vi "Continuity.vi"(0 "TSM context":T4, 5 "Supply Pins and Current Limits (set to 0V)":T1[](array[typedef]) {"Current Limit (A)" format="%#_13p"}, 7 "Continuity Test Pins and Current Levels":T3[](array[typedef]) {"Current Level (A)" format="%#_13p"}, 9 "Continuity Test Pins Configuration":T2={"DCPower Pins Voltage Limit (V)"=1.0, "Digital Pins Voltage Limit High (V)"=2.5, "Digital Pins Voltage Limit Low (V)"=-1.5, "Aperture Time (s)"=4e-06, "Settling Time (s)"=0.0005} {"Settling Time (s)" format="%#_13p"; "Aperture Time (s)" format="%#_13p"; "Digital Pins Voltage Limit Low (V)" format="%#_13p"; "Digital Pins Voltage Limit High (V)" format="%#_13p"; "DCPower Pins Voltage Limit (V)" format="%#_13p"}) -> (15 "error out":errorcluster)   [LabVIEW 2020]
doc: "This VI tests continuity on all DCPower or Digital pins specified in the input array. Continuity is tested serially for each pin by forcing the requested Test Level current, measuring and publishing the resulting voltage, and then forcing 0V on that line."
uses:
  <vilib>/NI_TestStand_SemiconductorModule/NI_TestStand_Semiconductor_Module.lvlibp/PinMap/General/SemiconductorModuleContext.ctl
  Typedefs/Continuity Test Pins.ctl
  Typedefs/Continuity Test Pins Configuration.ctl
  Typedefs/Continuity Test Supply Pins.ctl
  <vilib>/NI_TestStand_SemiconductorModule/NI_TestStand_Semiconductor_Module.lvlibp/PinMap/General/NIInstrumentTypeIDs.ctl
  <instrlib>/niDCPower/nidcpower.llb/niDCPower Sense.ctl
  <instrlib>/niDCPower/nidcpower.llb/niDCPower Wait For Event - Event.ctl
  69e15daa-21bc-4a86-876e-45ae4f872e77.vi
  7341af22-bb1b-4db6-ae5f-e70a74fc99ec.vi
  3f155922-c876-4283-947d-51e7db997094.vi
  cab31188-4031-40a5-8ba5-f7a05916ad31.vi
  4e72e363-04f0-4c76-a5e4-36f1355fad37.vi
  4a7f1c6e-2141-4ac2-bcbe-4ddac98e05b0.vi
  69e15daa-21bc-4a86-876e-45ae4f872e77.vi/37e36e8e-52ea-454a-87f9-b48a49eb94f9.vi
  69e15daa-21bc-4a86-876e-45ae4f872e77.vi/7a476e54-2186-4dad-b590-ad3942d096a6.vi
  69e15daa-21bc-4a86-876e-45ae4f872e77.vi/0fe00e69-3e59-4a7f-af61-7afbdd073a88.vi
  69e15daa-21bc-4a86-876e-45ae4f872e77.vi/e6b7bfbe-abe8-4733-8e43-b833ff7e14d5.vi
  7341af22-bb1b-4db6-ae5f-e70a74fc99ec.vi/e13535e0-0cde-4935-b31f-df609d882bf7.vi
  7341af22-bb1b-4db6-ae5f-e70a74fc99ec.vi/3a3479db-a9d1-451a-bc22-44f502cf356f.vi
  7341af22-bb1b-4db6-ae5f-e70a74fc99ec.vi/989d4714-5b7c-4079-81e3-211be10dc077.vi
  7341af22-bb1b-4db6-ae5f-e70a74fc99ec.vi/1a487ccc-7edf-462f-8e0a-db08c9486ef7.vi
  7341af22-bb1b-4db6-ae5f-e70a74fc99ec.vi/c9d031c9-6d94-47b7-9259-545c97247752.vi
  3f155922-c876-4283-947d-51e7db997094.vi/b53c6634-6278-4ab4-ad22-deef7c3257c8.vi
  3f155922-c876-4283-947d-51e7db997094.vi/c97d13a2-db54-44f2-8789-f416a58a5b16.vi
  3f155922-c876-4283-947d-51e7db997094.vi/975b8a18-37a4-405e-b68c-dfb8626d50ee.vi
  3f155922-c876-4283-947d-51e7db997094.vi/86300431-e79c-44d5-990a-071b252c0ae5.vi
  cab31188-4031-40a5-8ba5-f7a05916ad31.vi/9ed1208e-9e24-434b-9077-fc28cb587a19.vi
  cab31188-4031-40a5-8ba5-f7a05916ad31.vi/8ec5e351-fcbd-491e-9dc1-09518d2cf07d.vi
  cab31188-4031-40a5-8ba5-f7a05916ad31.vi/9a5011c0-d40c-4ff4-90a3-5e05d61ad4c8.vi
  cab31188-4031-40a5-8ba5-f7a05916ad31.vi/d089af44-28b1-43b8-9543-ae158de0acbd.vi
  4e72e363-04f0-4c76-a5e4-36f1355fad37.vi/ca0fc33b-5c63-48b0-b4a8-701cf7564698.vi
  4e72e363-04f0-4c76-a5e4-36f1355fad37.vi/d07ff0df-60b4-435a-afe9-5c803e6a7680.vi
  4e72e363-04f0-4c76-a5e4-36f1355fad37.vi/0037e193-eb15-4f67-9373-277439ca96e3.vi
  4e72e363-04f0-4c76-a5e4-36f1355fad37.vi/04a00edb-35d4-47ed-b21f-d8dfa56efb37.vi
  Common/Instrument Control/Digital/SubVIs/SSC Digital Calculate Per-Site Per-Pin to Per-Instrument LUT.vi
  4a7f1c6e-2141-4ac2-bcbe-4ddac98e05b0.vi/7ab91422-1a66-4814-9877-4eb2634f872c.vi
  4a7f1c6e-2141-4ac2-bcbe-4ddac98e05b0.vi/78867d26-a5ff-4ac0-84e1-08aa210c9386.vi
  3f155922-c876-4283-947d-51e7db997094.vi/86300431-e79c-44d5-990a-071b252c0ae5.vi/8c0f5037-9bd0-4b91-af38-cdea4b9b3604.vi
  Common/Instrument Control/Shared SubVIs/Trim Whitespace [Inlined].vi
  Common/Instrument Control/DCPower/SubVIs/SSC DCPower Expanded Pin List to SSC Index.vi
  Common/Instrument Control/Shared SubVIs/Channel List to Pins.vi
  <vilib>/NI_TestStand_SemiconductorModule/NI_TestStand_Semiconductor_Module.lvlibp/PinMap/PinQueryContext/MultiplePinMultipleSessionQueryContext/MultiplePinMultipleSessionQueryContext.lvclass
  C:/Program Files/National Instruments/LabVIEW 2020/vi.lib/NI_TestStand_SemiconductorModule/NI_TestStand_Semiconductor_Module.lvlibp/PinMap/PinQueryContext/PinQueryContext.lvclass
  <vilib>/NI_TestStand_SemiconductorModule/NI_TestStand_Semiconductor_Module.lvlibp/PinMap/Digital Pattern/PinQueryContext/DigitalPatternPinQueryContext.lvclass
  C:/Program Files/National Instruments/LabVIEW 2020/vi.lib/NI_TestStand_SemiconductorModule/NI_TestStand_Semiconductor_Module.lvlibp/PinMap/PinQueryContext/MultipleSessionPinQueryContext.lvclass
  Common/Instrument Control/Digital/SSC Digital/PPMU/SSC Digital PPMU Source Voltage.vi
  Common/Instrument Control/DCPower/SSC DCPower/Source/Constant Voltage/SSC DCPower Force Voltage Array Symmetric Limits.vi
  Common/Instrument Control/DCPower/SSC DCPower/SSC DCPower Configure Measurements.vi
  Common/Instrument Control/DCPower/SSC DCPower/Measure/SSC DCPower Configure Settings Array.vi
  <vilib>/Utility/error.llb/Error Cluster From Error Code.vi
  Common/Instrument Control/Digital/SSC Digital/PPMU/SSC Digital PPMU Configure Voltage Limits.vi
  Common/Instrument Control/Digital/SSC Digital/PPMU/SSC Digital PPMU Configure Aperture Time.vi
  Common/Instrument Control/DCPower/SSC DCPower/Source/Constant Current/SSC DCPower Force Current Array Symmetric Limits.vi
  Common/Instrument Control/DCPower/SSC DCPower/Triggers and Events/SSC DCPower Wait for Event.vi
  Common/Instrument Control/DCPower/SSC DCPower/SSC DCPower Measure.vi
  <vilib>/NI_TestStand_SemiconductorModule/NI_TestStand_Semiconductor_Module.lvlibp/PinMap/General/Publish/PublishDataDouble1D.vi
  Common/Instrument Control/Digital/SSC Digital/PPMU/SSC Digital PPMU Source Current.vi
  <vilib>/NI_TestStand_SemiconductorModule/NI_TestStand_Semiconductor_Module.lvlibp/PinMap/General/Publish/PublishDataDouble2D.vi
  <vilib>/NI_TestStand_SemiconductorModule/NI_TestStand_Semiconductor_Module.lvlibp
  C:/Program Files/National Instruments/LabVIEW 2020/vi.lib/NI_TestStand_SemiconductorModule/NI_TestStand_Semiconductor_Module.lvlibp/PinMap/PinQueryContext/MultiplePinMultipleSessionQueryContext/MultiplePinMultipleSessionQueryContext.lvclass
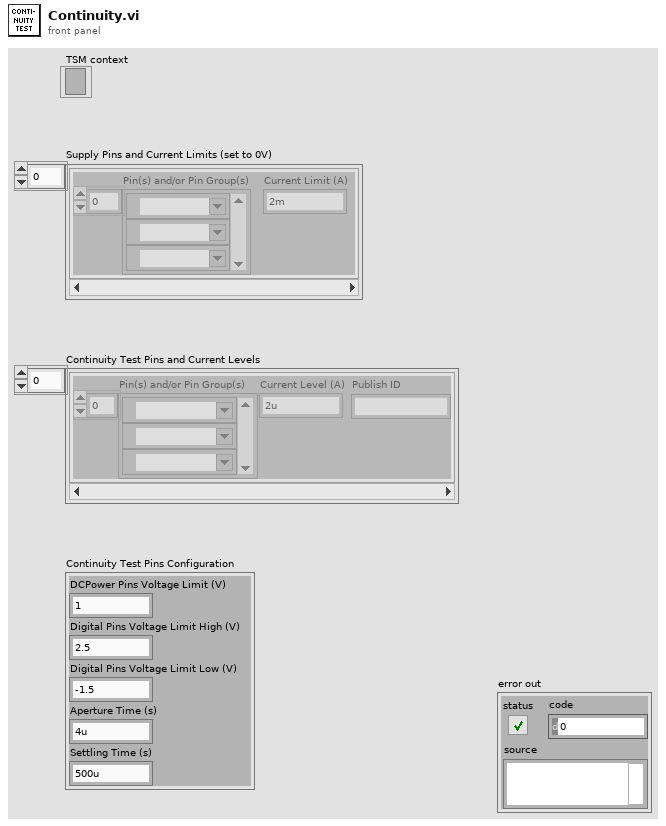
[diagram p1: front panel]
types:
  T1 = typedef "Continuity Test Supply Pins.ctl" = cluster{"Pin(s) and/or Pin Group(s)":tag[], "Current Limit (A)":dbl}
  T2 = typedef "Continuity Test Pins Configuration.ctl" = cluster{"DCPower Pins Voltage Limit (V)":dbl, "Digital Pins Voltage Limit High (V)":dbl, "Digital Pins Voltage Limit Low (V)":dbl, "Aperture Time (s)":dbl, "Settling Time (s)":dbl}
  T3 = typedef "Continuity Test Pins.ctl" = cluster{"Pin(s) and/or Pin Group(s)":tag[], "Current Level (A)":dbl, "Publish ID":string}
  T4 = typedef "NI_TestStand_Semiconductor_Module.lvlibp/SemiconductorModuleContext.ctl" = refnum<k7>
  T5 = cluster{"Site Numbers":i32[], "DCPower Test Levels (A)":dbl[], "DCPower Test Pins":tag[], "DCPower Publish IDs":tag[], "Digital Test Levels (A)":dbl[], "Digital Test Pins":tag[], "Digital Publish IDs":tag[], "Digital Current Range (A)":dbl}
  T6 = typedef "NI_TestStand_Semiconductor_Module.lvlibp/NIInstrumentTypeIDs.ctl" = string
  T7 = typedef "NI_TestStand_Semiconductor_Module.lvlibp/TSM_Pin.ctl" = tag
  T8 = typedef "TSM SSC Digital.ctl" = cluster{"Pin Query Context":refnum<class "DigitalPatternPinQueryContext.lvclass">, "SSC":T9[], "Site Numbers":i32[], "Pins":tag[]}
  T9 = typedef "SSC Digital.ctl" = cluster{"Session":refnum<k15>, "Channel List":string, "Site List":string}
  T10 = typedef "TSM SSC DCPower.ctl" = cluster{"Pin Query Context":refnum<class "MultiplePinMultipleSessionQueryContext.lvclass">, "SSC":T11[], "Site Numbers":i32[], "Pins":T12[], "Pins Expanded":T14[]}
  T11 = typedef "SSC DCPower.ctl" = cluster{"Session":refnum<k15>, "Chan":string, "Channel List":string}
  T12 = typedef "TSM Pin Information.ctl" = cluster{"Pin":tag, "Type":T13, "Count":i32}
  T13 = typedef "TSM Pin Type Identifier.ctl" = enum8{"DUT Pin", "System Pin", "Pin Group", "Not Determined"}
  T14 = typedef "TSM Expanded Pin Information.ctl" = cluster{"Pin":tag, "Type":T13, "Index":i32}
  T15 = typedef "niDCPower Sense.ctl" = i32
  T16 = typedef "niDCPower Wait For Event - Event.ctl" = i32
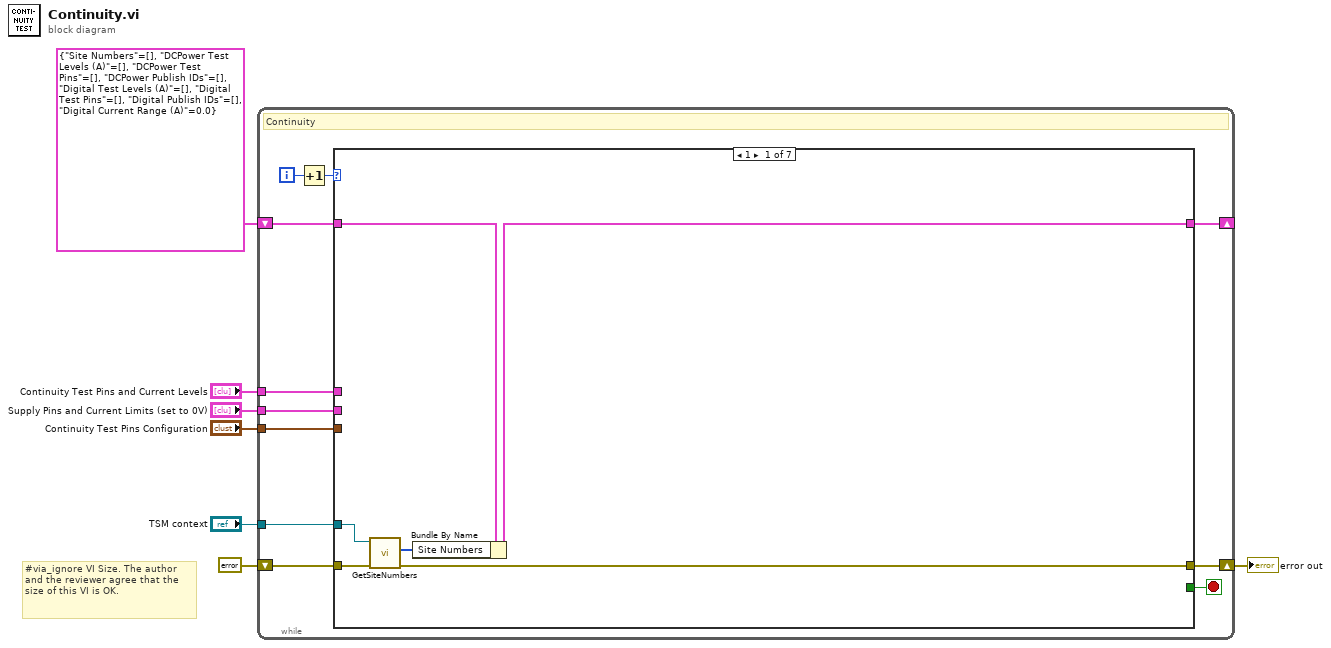
[diagram p0: block diagram]
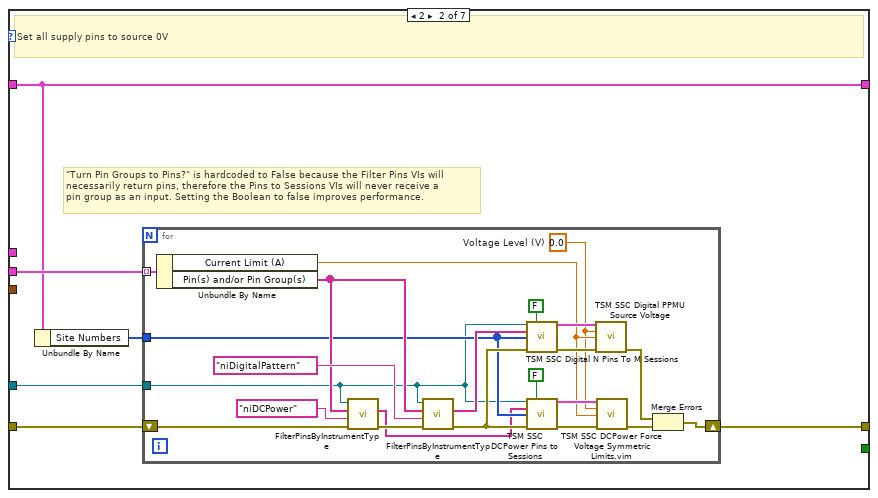
[diagram p2: hidden frame]
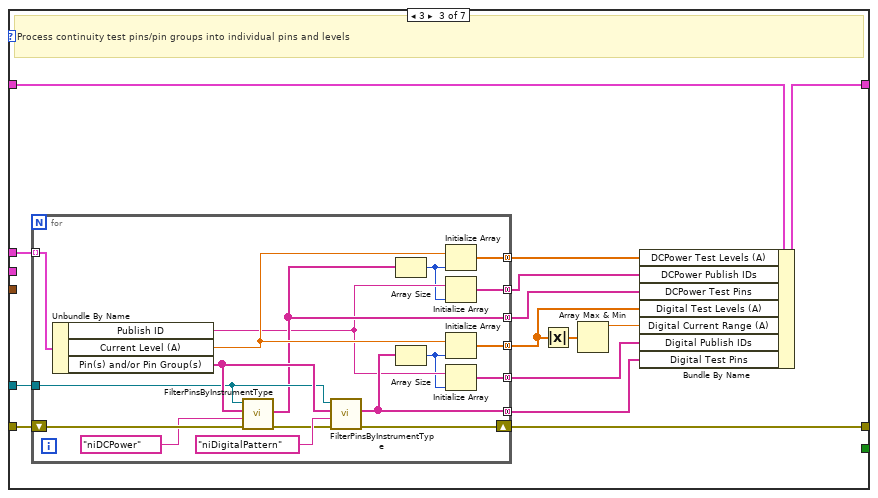
[diagram p3: hidden frame]
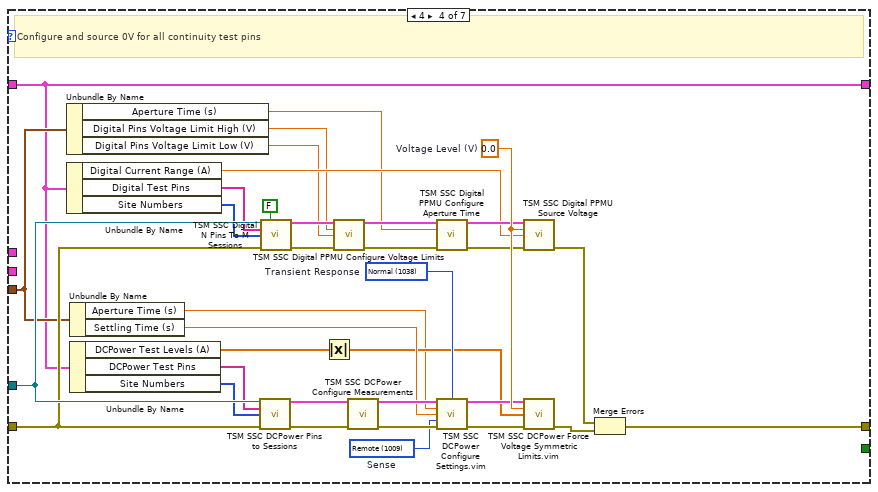
[diagram p4: hidden frame]
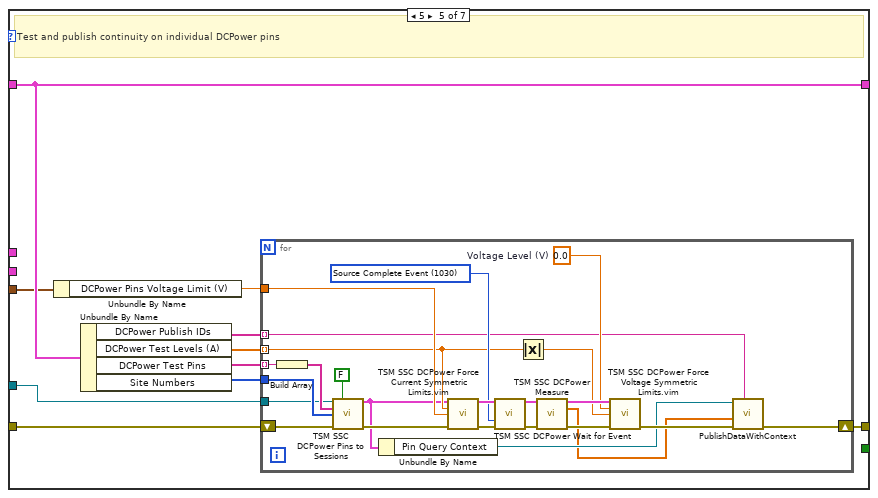
[diagram p5: hidden frame]
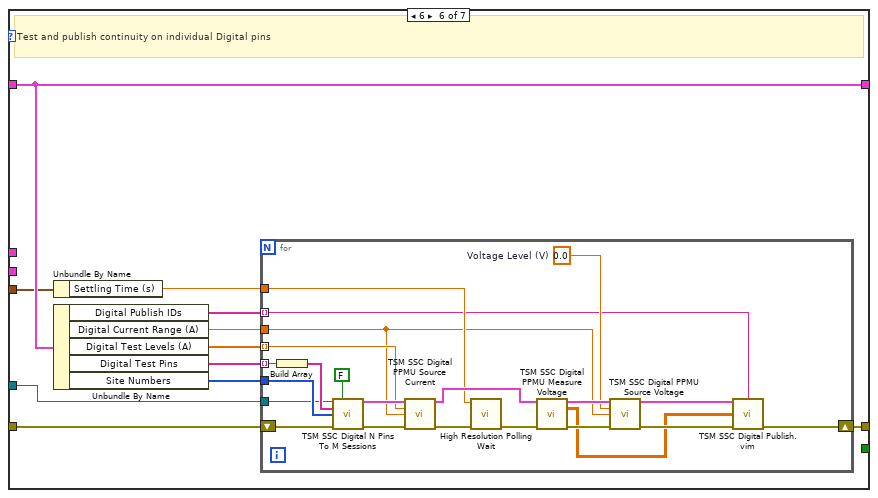
[diagram p6: hidden frame]
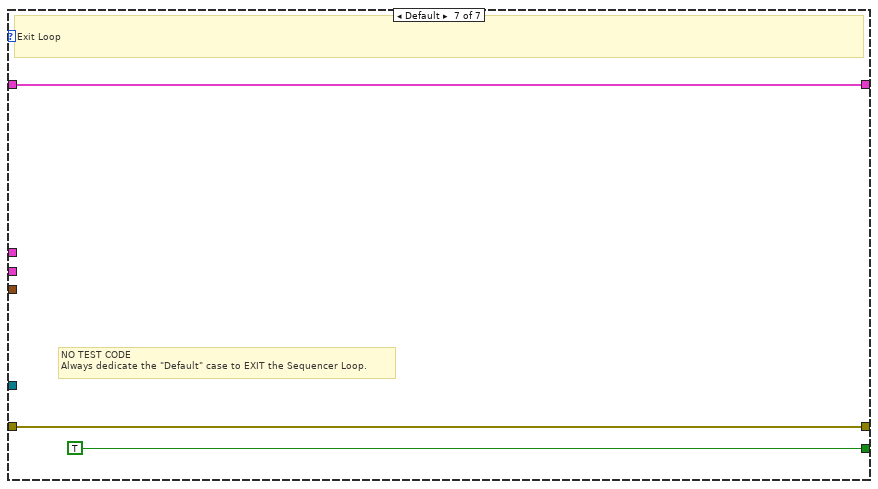
[diagram p7: hidden frame]
diagram:
  # "#via_ignore VI Size. The author and the reviewer agree that the size of this VI is OK."
  n1 = while {
    shift-right: [w16] -> w7
    shift-left: errorcluster {"status"=FALSE, "code"=0, "source"=""} ("error in") -> [w17]
    tunnel: "TSM context" -> [w14]
    shift-right: [w11] -> _
    shift-left: T5 {"Site Numbers"=[], "DCPower Test Levels (A)"=[], "DCPower Test Pins"=[], "DCPower Publish IDs"=[], "Digital Test Levels (A)"=[], "Digital Test Pins"=[], "Digital Publish IDs"=[], "Digital Current Range (A)"=0.0} -> [w12]
    tunnel: "Supply Pins and Current Limits (set to 0V)" -> [w10]
    tunnel: "Continuity Test Pins and Current Levels" -> [w9]
    tunnel: "Continuity Test Pins Configuration" -> [w8]
    i -> [w18]
    stop <- w13 stop-if-true
    # "Continuity"
    n2 = Increment(x=w18) -> (x+1=w15:i32)
    n3 = case shown="1" w15 {
      tunnel: [w21 w27 w64 w99 w128 w163 w188] -> w16
      tunnel: w17 -> [w23 w30 w65 w97 w129 w164 w188]
      tunnel: w14 -> [w22 w28 w63 w118 w123 w158 _]
      tunnel: [_ _ _ _ _ _ TRUE] -> w13
      tunnel: w12 -> [w19 w26 w66 w89 w127 w162 w187]
      tunnel: [w20 w26 w61 w89 w127 w162 w187] -> w11
      tunnel: w10 -> [_ w29 _ _ _ _ _]
      tunnel: w9 -> [_ _ w62 _ _ _ _]
      tunnel: w8 -> [_ _ _ w95 w122 w157 _]
      frame 1 {
        n4 = call <vilib>:"GetSiteNumbers.vi"("error in (no error)"=w23, "Semiconductor Module Context"=w22) -> ("error out"=w21:errorcluster, "Site Numbers"=w24:i32[])  [unwired: 6 in, 2 out]
        n5 = Bundle By Name(cluster=w19, "Site Numbers"=w24) -> (w20:T5)
      }
      frame 2 {
        # "\"Turn Pin Groups to Pins?\" is hardcoded to False because the Filter Pins VIs will\nnecessarily return pins, therefore the Pins to Sessions VIs will never receive a \npin group as an input. Setting the Boolean to false improves performance."
        # "Set all supply pins to source 0V"
        n6 = Unbundle By Name(w26) -> ("Site Numbers"=w25:i32[])
        n7 = for {
          shift-right: [w51] -> w27
          shift-left: w30 -> [w52]
          tunnel: w29 -> [w48] mode=indexing
          tunnel: w28 -> [w31]
          tunnel: w25 -> [w33]
          w39 = 0.0  # Voltage Level (V)
          n8 = Unbundle By Name(w48) -> ("Current Limit (A)"=w40:dbl, "Pin(s) and/or Pin Group(s)"=w47:tag[])
          n9 = call <vilib>:"FilterPinsByInstrumentType.vi"("error in (no error)"=w52, "Instrument Type Id"=T6 "niDCPower", "Pins"=w47, "Semiconductor Module Context"=w31) -> ("error out"=w36:errorcluster, "Filtered Pins"=w32:T7[])  [unwired: 5 in, 1 out]
          n10 = call <vilib>:"FilterPinsByInstrumentType.vi"("error in (no error)"=w36, "Instrument Type Id"=T6 "niDigitalPattern", "Pins"=w47, "Semiconductor Module Context"=w31) -> ("error out"=w35:errorcluster, "Filtered Pins"=w34:T7[])  [unwired: 5 in, 1 out]
          n11 = call "TSM SSC Digital N Pins To M Sessions.vi"("TSM context"=w31, "Turn Pin Groups to Pins?"=FALSE ("Turn Pin Groups to Pins? (T)"), "Pins"=w34, "Site Numbers"=w33, "error in"=w35) -> ("Digital TSM Out"=w43:T8, "error out"=w46:errorcluster)  [unwired: 9 in]
          n12 = call "TSM SSC DCPower Pins to Sessions.vi"("TSM context"=w31, "Fill SSC Pin and Site Information? (T)"=FALSE ("Turn Pin Groups to Pins? (F)"), "Pins"=w32, "Site Numbers"=w33, "error in"=w35) -> ("DCPower TSM Out"=w41:T10, "error out"=w45:errorcluster)  [unwired: 9 in]
          n13 = call "TSM SSC Digital PPMU Source Voltage.vi"("Digital TSM In"=w43, "Voltage Level (V)"=w39, "Current Limit Range (A)"=w40, "error in"=w46) -> ("error out"=w44:errorcluster)  [unwired: 10 in, 1 out]
          n14 = call "TSM SSC DCPower Force Voltage Symmetric Limits.vim"("DCPower TSM in"=w41, "Voltage Level (V)"=w39, "Current Limit (A)"=w40, "error in"=w45) -> ("error out"=w42:errorcluster)  [unwired: 10 in, 1 out]
          n15 = Merge Errors(w44, w42) -> (w51:errorcluster)
        }
      }
      frame 3 {
        # "Process continuity test pins/pin groups into individual pins and levels"
        n16 = for {
          shift-right: [w76] -> w64
          shift-left: w65 -> [w84]
          tunnel: w63 -> [w81]
          tunnel: w62 -> [w80] mode=indexing
          tunnel: [w75] -> w60 mode=concatenating
          tunnel: [w74] -> w56 mode=concatenating
          tunnel: [w73] -> w59 mode=concatenating
          tunnel: [w72] -> w55 mode=concatenating
          tunnel: [w68] -> w54 mode=concatenating
          tunnel: [w67] -> w53 mode=concatenating
          n17 = Unbundle By Name(w80) -> ("Publish ID"=w71:string, "Current Level (A)"=w77:dbl, "Pin(s) and/or Pin Group(s)"=w82:tag[])
          n18 = call <vilib>:"FilterPinsByInstrumentType.vi"("error in (no error)"=w84, "Instrument Type Id"=T6 "niDCPower", "Pins"=w82, "Semiconductor Module Context"=w81) -> ("error out"=w78:errorcluster, "Filtered Pins"=w74:T7[])  [unwired: 5 in, 1 out]
          n19 = call <vilib>:"FilterPinsByInstrumentType.vi"("error in (no error)"=w78, "Instrument Type Id"=T6 "niDigitalPattern", "Pins"=w82, "Semiconductor Module Context"=w81) -> ("error out"=w76:errorcluster, "Filtered Pins"=w72:T7[])  [unwired: 5 in, 1 out]
          n20 = Array Size(array=w74) -> (size(s)=w70:i32)
          n21 = Array Size(array=w72) -> (size(s)=w69:i32)
          n22 = Initialize Array(w77, w70) -> (w75:dbl[])
          n23 = Initialize Array(w71, w70) -> (w67:string[])
          n24 = Initialize Array(w77, w69) -> (w73:dbl[])
          n25 = Initialize Array(w71, w69) -> (w68:string[])
        }
        n26 = Absolute Value(x=w59) -> (abs(x)=w57:dbl[])
        n27 = Array Max & Min(array=w57) -> (max value=w58:dbl)  [unwired: 3 out]
        n28 = Bundle By Name(cluster=w66, "DCPower Test Levels (A)"=w60, "DCPower Publish IDs"=w53, "DCPower Test Pins"=w56, "Digital Test Levels (A)"=w59, "Digital Current Range (A)"=w58, "Digital Publish IDs"=w54, "Digital Test Pins"=w55) -> (w61:T5)
      }
      frame 4 {
        w106 = 1038 items=["Slow"=1041, "Normal"=1038, "Fast"=1039, "Custom"=1042]  # Transient Response
        w107 = T15 1009 items=["Local"=1008, "Remote"=1009]  # Sense
        w114 = 0.0  # Voltage Level (V)
        # "Configure and source 0V for all continuity test pins"
        n29 = Unbundle By Name(w95) -> ("Aperture Time (s)"=w86:dbl, "Digital Pins Voltage Limit High (V)"=w88:dbl, "Digital Pins Voltage Limit Low (V)"=w87:dbl)
        n30 = Unbundle By Name(w89) -> ("Digital Current Range (A)"=w100:dbl, "Digital Test Pins"=w117:tag[], "Site Numbers"=w91:i32[])
        n31 = Unbundle By Name(w95) -> ("Aperture Time (s)"=w94:dbl, "Settling Time (s)"=w108:dbl)
        n32 = Unbundle By Name(w89) -> ("DCPower Test Levels (A)"=w96:dbl[], "DCPower Test Pins"=w93:tag[], "Site Numbers"=w92:i32[])
        n33 = call "TSM SSC DCPower Pins to Sessions.vi"("TSM context"=w118, "Pins"=w93, "Site Numbers"=w92, "error in"=w97) -> ("DCPower TSM Out"=w85:T10, "error out"=w119:errorcluster)  [unwired: 10 in]
        n34 = call "TSM SSC Digital N Pins To M Sessions.vi"("TSM context"=w118, "Turn Pin Groups to Pins?"=FALSE ("Turn Pin Groups to Pins? (T)"), "Pins"=w117, "Site Numbers"=w91, "error in"=w97) -> ("Digital TSM Out"=w103:T8, "error out"=w102:errorcluster)  [unwired: 9 in]
        n35 = Absolute Value(x=w96) -> (abs(x)=w101:dbl[])
        n36 = call "TSM SSC Digital PPMU Configure Voltage Limits.vi"("Digital TSM In"=w103, "Voltage Limit High (V)"=w88, "Voltage Limit Low (V)"=w87, "error in"=w102) -> ("Digital TSM Out"=w113:T8, "error out"=w115:errorcluster)  [unwired: 10 in]
        n37 = call "TSM SSC DCPower Configure Measurements.vi"("DCPower SSC in"=w85, "error in"=w119) -> ("DCPower SSC out"=w110:T10, "error out"=w112:errorcluster)  [unwired: 12 in]
        n38 = call "TSM SSC Digital PPMU Configure Aperture Time.vi"("Digital TSM In"=w113, "Aperture Time (s)"=w86, "error in"=w115) -> ("Digital TSM Out"=w104:T8, "error out"=w105:errorcluster)  [unwired: 11 in]
        n39 = call "TSM SSC DCPower Configure Settings.vim"("DCPower TSM in"=w110, "Transient Response"=w106, "Aperture Time"=w94, "Source Delay (s)"=w108, "Sense"=w107, "error in"=w112) -> ("DCPower TSM out"=w109:T10, "error out"=w111:errorcluster)  [unwired: 8 in]
        n40 = call "TSM SSC Digital PPMU Source Voltage.vi"("Digital TSM In"=w104, "Voltage Level (V)"=w114, "Current Limit Range (A)"=w100, "error in"=w105) -> ("error out"=w98:errorcluster)  [unwired: 10 in, 1 out]
        n41 = call "TSM SSC DCPower Force Voltage Symmetric Limits.vim"("DCPower TSM in"=w109, "Voltage Level (V)"=w114, "Current Limit (A)"=w101, "error in"=w111) -> ("error out"=w116:errorcluster)  [unwired: 10 in, 1 out]
        n42 = Merge Errors(w98, w116) -> (w99:errorcluster)
      }
      frame 5 {
        # "Test and publish continuity on individual DCPower pins"
        n43 = Unbundle By Name(w122) -> ("DCPower Pins Voltage Limit (V)"=w121:dbl)
        n44 = Unbundle By Name(w127) -> ("DCPower Publish IDs"=w120:tag[], "DCPower Test Levels (A)"=w124:dbl[], "DCPower Test Pins"=w125:tag[], "Site Numbers"=w126:i32[])
        n45 = for {
          shift-right: [w148] -> w128
          shift-left: w129 -> [w153]
          tunnel: w126 -> [w146]
          tunnel: w125 -> [w145] mode=indexing
          tunnel: w124 -> [w135] mode=indexing
          tunnel: w123 -> [w143]
          tunnel: w121 -> [w138]
          tunnel: w120 -> [w132] mode=indexing
          w136 = 0.0  # Voltage Level (V)
          w137 = T16 1030 items=["Source Complete Event"=1030, "Measure Complete Event"=1031, "Sequence Iteration Complete Event"=1032, "Sequence Engine Done Event"=1033, "Pulse Complete Event"=1051, "Ready For Pulse Trigger Event"=1052] ("Event")
          n46 = Build Array(w145) -> (w144:tag[])
          n47 = call "TSM SSC DCPower Pins to Sessions.vi"("TSM context"=w143, "Fill SSC Pin and Site Information? (T)"=FALSE ("Turn Pin Groups to Pins? (F)"), "Pins"=w144, "Site Numbers"=w146, "error in"=w153) -> ("DCPower TSM Out"=w130:T10, "error out"=w147:errorcluster)  [unwired: 9 in]
          n48 = Unbundle By Name(w130) -> ("Pin Query Context"=w139:refnum<class "MultiplePinMultipleSessionQueryContext.lvclass">)
          n49 = call "TSM SSC DCPower Force Current Symmetric Limits.vim"("DCPower TSM in"=w130, "Current Level (A)"=w135, "Voltage Limit (V)"=w138, "error in"=w147) -> ("DCPower TSM out"=w142:T10, "error out"=w152:errorcluster)  [unwired: 10 in]
          n50 = call "TSM SSC DCPower Wait for Event.vi"("DCPower TSM in"=w142, "Event"=w137, "error in"=w152) -> ("DCPower TSM out"=w141:T10, "error out"=w150:errorcluster)  [unwired: 11 in]
          n51 = Absolute Value(x=w135) -> (abs(x)=w133:dbl)
          n52 = call "TSM SSC DCPower Measure.vi"("DCPower TSM in"=w141, "error in"=w150) -> ("DCPower TSM out"=w140:T10, "Voltage Measurements (V)"=w131:dbl[], "error out"=w149:errorcluster)  [unwired: 10 in, 1 out]
          n53 = call "TSM SSC DCPower Force Voltage Symmetric Limits.vim"("DCPower TSM in"=w140, "Voltage Level (V)"=w136, "Current Limit (A)"=w133, "error in"=w149) -> ("error out"=w151:errorcluster)  [unwired: 10 in, 1 out]
          n54 = call-poly <vilib>:"PublishDataWithContext.vi"("Published Data Id"=w132, "error in (no error)"=w151, "Data In"=w131, "Pin Query Context"=w139) -> ("error out"=w148:errorcluster)  [unwired: 6 in, 1 out]
        }
      }
      frame 6 {
        # "Test and publish continuity on individual Digital pins"
        n55 = Unbundle By Name(w157) -> ("Settling Time (s)"=w156:dbl)
        n56 = Unbundle By Name(w162) -> ("Digital Publish IDs"=w154:tag[], "Digital Current Range (A)"=w155:dbl, "Digital Test Levels (A)"=w159:dbl[], "Digital Test Pins"=w160:tag[], "Site Numbers"=w161:i32[])
        n57 = for {
          shift-right: [w181] -> w163
          shift-left: w164 -> [w186]
          tunnel: w161 -> [w179]
          tunnel: w160 -> [w178] mode=indexing
          tunnel: w159 -> [w167] mode=indexing
          tunnel: w158 -> [w176]
          tunnel: w156 -> [w168]
          tunnel: w155 -> [w166]
          tunnel: w154 -> [w165] mode=indexing
          w173 = 0.0  # Voltage Level (V)
          n58 = Build Array(w178) -> (w177:tag[])
          n59 = call "TSM SSC Digital N Pins To M Sessions.vi"("TSM context"=w176, "Turn Pin Groups to Pins?"=FALSE ("Turn Pin Groups to Pins? (T)"), "Pins"=w177, "Site Numbers"=w179, "error in"=w186) -> ("Digital TSM Out"=w171:T8, "error out"=w180:errorcluster)  [unwired: 9 in]
          n60 = call "TSM SSC Digital PPMU Source Current.vi"("Digital TSM In"=w171, "Current Level (A)"=w167, "Current Level Range (A)"=w166, "error in"=w180) -> ("Digital TSM Out"=w170:T8, "error out"=w185:errorcluster)  [unwired: 10 in]
          n61 = call <vilib>:"High Resolution Polling Wait.vi"("error in (no error)"=w185, "seconds to wait"=w168) -> ("error out"=w183:errorcluster)  [unwired: 9 in]
          n62 = call "TSM SSC Digital PPMU Measure Voltage.vi"("Digital TSM In"=w170, "error in"=w183) -> ("Digital TSM Out"=w175:T8, "Per-Site Per-Pin Measurements (V)"=w174:dbl[][], "error out"=w182:errorcluster)  [unwired: 11 in]
          n63 = call "TSM SSC Digital PPMU Source Voltage.vi"("Digital TSM In"=w175, "Voltage Level (V)"=w173, "Current Limit Range (A)"=w166, "error in"=w182) -> ("Digital TSM Out"=w169:T8, "error out"=w184:errorcluster)  [unwired: 10 in]
          n64 = call "TSM SSC Digital Publish.vim"("Digital TSM In"=w169, "Published Data Id"=w165, "Data to Publish"=w174, "error in (no error)"=w184) -> ("error out"=w181:errorcluster)  [unwired: 10 in, 1 out]
        }
      }
      frame Default {
        # "NO TEST CODE\nAlways dedicate the \"Default\" case to EXIT the Sequencer Loop."
        # "Exit Loop"
      }
    }
  }
  "error out" <- w7
